vi "Halvorsen_IMP_SVI.vi"(0 "Шаг h, с":ext, 1 "n":i32[](array[numeric]), 2 "k":i32, 3 "Parameter_Vector":ext[](array[numeric]), 5 "Время, с":ext, 7 "Initial Conditions":ext[](array[numeric]), 9 "Hmin":ext, 12 "Hmax":ext, 13 "tolerance":ext) -> (4 "Solution":ext[][](array[numeric]))   [LabVIEW 2016]
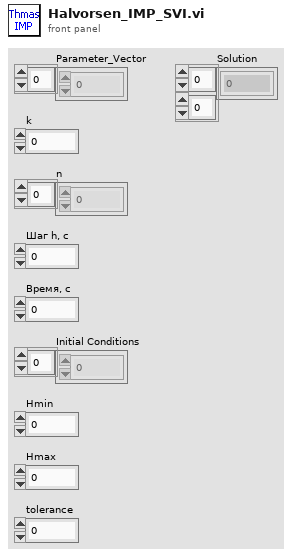
[diagram p1: front panel]
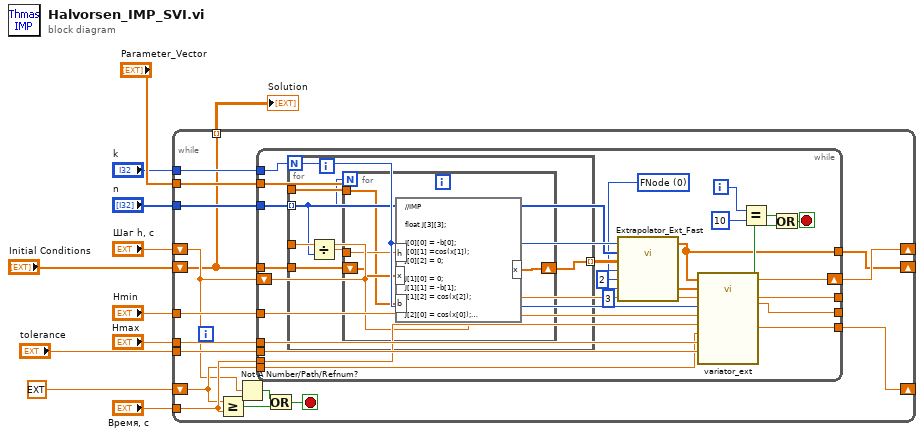
[diagram p0: block diagram]
diagram:
  n1 = while {
    shift-right: [w21] -> _
    shift-left: "Initial Conditions" -> [w12]
    tunnel: "n" -> [w27]
    tunnel: "k" -> [w26]
    shift-right: [w22] -> _
    shift-left: "Шаг h, с" -> [w14]
    shift-right: [w18] -> _
    shift-left: ext 0.0 -> [w19]
    tunnel: "Время, с" -> [w20]
    tunnel: "tolerance" -> [w23]
    tunnel: "Hmin" -> [w25]
    tunnel: "Hmax" -> [w24]
    tunnel: [w12] -> w9 mode=indexing
    tunnel: "Parameter_Vector" -> [w17]
    stop <- w16 stop-if-true
    n2 = Greater Or Equal?(x=w19, y=w20) -> (x >= y?=w15:bool)
    n3 = Not A Number/Path/Refnum?(number/path/refnum=w14) -> (NaN/Path/Refnum?=w13:bool)
    n4 = while {
      tunnel: w25 -> [w44]
      tunnel: w24 -> [w49]
      tunnel: w23 -> [w43]
      tunnel: w26 -> [w47]
      tunnel: w27 -> [w46]
      tunnel: w12 -> [w45]
      shift-right: [w38] -> w22
      shift-left: w14 -> [w30]
      tunnel: [w30] -> _
      tunnel: [w37] -> _
      tunnel: [w36] -> w21
      tunnel: w20 -> [w35]
      tunnel: w19 -> [w34]
      tunnel: [w32] -> w18
      tunnel: w17 -> [w31]
      i -> [w33]
      stop <- w39 stop-if-true
      w28 = u16 0 items=["FNode", "MathScript", "ECD8 Arrays", "ECD8 Fnode", "ECD8 FnodeDiv"] ("Ext.Type")
      n5 = for {
        N: w47 -> [_]
        tunnel: w46 -> [w52] mode=indexing
        tunnel: w30 -> [w57]
        tunnel: w45 -> [w55]
        tunnel: [w56] -> w48 mode=indexing
        tunnel: w31 -> [w53]
        n6 = Divide(x=w57, y=w52) -> (x/y=w54:ext)
        n7 = for {
          N: w52 -> [_]
          shift-right: [w61] -> w56
          shift-left: w55 -> [w60]
          tunnel: w54 -> [w59]
          tunnel: w53 -> [w58]
          n8 = formula code="//IMP\n\nfloat J[3][3];\n\nJ[0][0] = -b[0]; \nJ[0][1] =cos(x[1]); \nJ[0][2] = 0; \n\nJ[1][0] = 0; \nJ[1][1] = -b[1];\nJ[1][2] = cos(x[2]);\n\nJ[2][0] = cos(x[0]); \nJ[2][1] =0;\nJ[2][2] = -b[2];\n\n\nfloat w[3][4], Z[3], a[3], Zn[3], dz;\nfloat tol;\nint k; int i; int j; float t; float d;\ntol = 1e-14;\nint nnewtmax = 3, nnewt;\ndz = 2e-13;\nnnewt = 0;\n\nZ[0] = x[0]; Z[1] = x[1]; Z[2] = x[2];\nwhile ( (dz > tol) && (nnewt < nnewtmax)){\n\nfor(i=0;i<3;i++){\nfor(j=0;j<3;j++){\nif (i==j)\nw[i][j]=1 - 0.5*h*J[i][j];\nelse\nw[i][j]= - 0.5*h*J[i][j];\n}}\n\n\n\na[0] = 0.5*(x[0] + Z[0]);\na[1] = 0.5*(x[1] + Z[1]);\na[2] = 0.5*(x[2] + Z[2]);\n\n\n\nw[0][3]=-Z[0]+x[0]+h*(-b[0]*a[0]+sin(a[1]));\nw[1][3]= -Z[1]+x[1]+h*(-b[1]*a[1]+sin(a[2]));\nw[2][3]= -Z[2]+x[2]+h*(-b[2]*a[2]+sin(a[0]));\n\n\nfor(k = 0; k <= 1; k++){\n\tint l = k;\n\n\tfor( i = k+1; i<= 2; i++){\n\t\tif( abs(w[i][k]) > abs(w[l][k]) ){\n\t\t\tl = i;\n\t\t}\n\t}\n\tif (l != k){\n\t\tfor( j = 0; j <= 3; j++){\n\t\t\tif ((j == 0) || (j >= k)){\n\t\t\t\tt = w[k][j];\n\t\t\t\tw[k][j] = w[l][j];\n\t\t\t\tw[l][j] = t;\n\t\t\t}\n\t\t}\n\t}\t\n\n\td = 1.0 / w[k][k];\n\tfor( i=(k+1); i <=(2); i++){\n\t\tif (w[i][k] == 0){\n\t\t\tcontinue;\n\t\t}\n\t\tt = w[i][k] * d;\n\t\tfor ( j = k; j <= (3); j++) {\n\t\t\tif (w[k][j] != 0){\n\t\t\t\tw[i][j] = w[i][j] - t * w[k][j];\n\t\t\t}\n\t\t}\n\t}\n}\nfor( i=(3); i >= 2; i--){\n\tfor( j=1; j <= i-1; j++){\n\t\tt = w[i - j - 1][i - 1]/w[ i -1][i - 1];\n\t\tw[i-j - 1][ 3] = w[i-j -1][3] - t*w[i - 1][ 3];\n\t}\n\tw[i-1][ 3] = w[i - 1][3]/w[ i -1][i - 1];\n}\nw[0][3] = w[0][3]/w[0][0];\nZn[0] = Z[0]+ w[0][3];\nZn[1] = Z[1]+ w[1][3];\nZn[2] = Z[2]+ w[2][3];\n\ndz = ( (Zn[0] - Z[0])**2 + (Zn[1] - Z[1])**2 + (Zn[2] - Z[2])**2 )**0.5;\nZ[0] = Zn[0];\nZ[1] = Zn[1];\nZ[2] = Zn[2];\n\n\nnnewt ++;\n}\n\nx[0] = Zn[0];\nx[1] = Zn[1];\nx[2] = Zn[2];"("x"=w60, "b"=w58, "h"=w59) -> ("x"=w61:ext[])
        }
      }
      n9 = call "Extrapolator_Ext_Fast.vi"("Порядок экстраполятора"=2 ("Ext. Order"), "Dimension"=3 ("input variable"), "Ext.Type"=w28, "Х - нач. условия"=w48, "n"=w46, "k"=w47) -> ("TPrev"=w50:ext[], "Tout"=w36:ext[])  [unwired: 4 in]
      n10 = call "variator_ext.vi"("Tout"=w36, "tolerance"=w43, "Hmax"=w49, "TPrev"=w50, "Шаг h, с"=w30, "Current time"=w34, "k"=w47, "Hmin"=w44, "tmax"=w35) -> ("Hnew"=w38:ext, "error estimation"=w37:ext, "New time"=w32:ext, "stop"=w40:bool)  [unwired: 3 in]
      n11 = Equal?(x=w33, y=10) -> (x = y?=w41:bool)
      n12 = Or(x=w41, y=w40) -> (x .or. y?=w39:bool)
    }
    n13 = Or(x=w13, y=w15) -> (x .or. y?=w16:bool)
  }
  "Solution" <- w9
